vi "Support_CheckLogCallOrder.vi"(2 "log":T1[](array[typedef]) {"timestamp" format="%<%H:%M:%S%2u\n%Y/%m/%d>T"}, 3 "Wanted call order VIs":string[](array[string]), 5 "error in (no error)":errorcluster, 7 "start index":i32, 9 "length":i32=-1) -> (16 "Correct call order?":bool, 19 "error out":errorcluster)   [LabVIEW 2009]
doc: "Checks if wanted call order is same as logged call order."
uses:
  Support_LogType.ctl
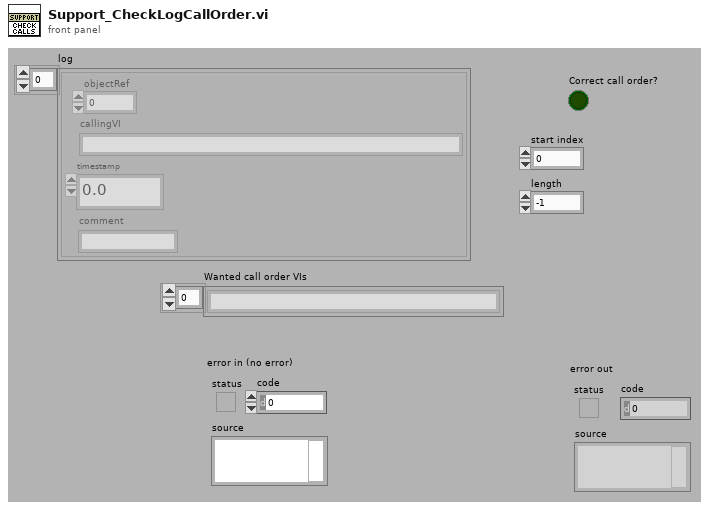
[diagram p1: front panel]
types:
  T1 = typedef "Support_LogType.ctl" = cluster{"objectRef":i32, "callingVI":string, "timestamp":dbl, "comment":string}
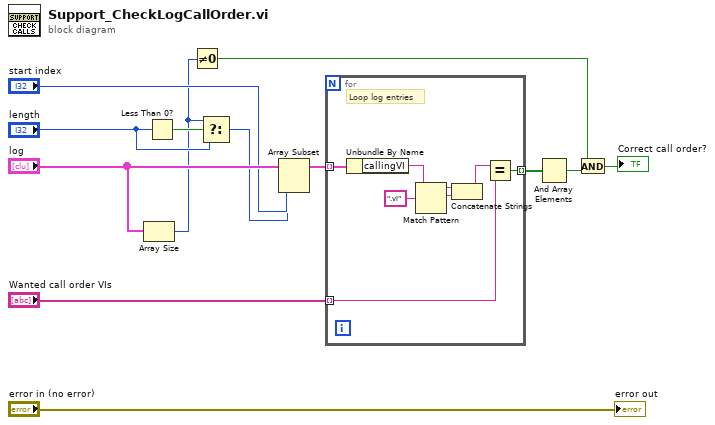
[diagram p0: block diagram]
diagram:
  n1 = Array Size(array="log") -> (size(s)=w4:i32)
  n2 = Less Than 0?(x="length") -> (x < 0?=w10:bool)
  n3 = Not Equal To 0?(x=w4) -> (x != 0?=w1:bool)
  n4 = Select(t=w4, s=w10, f="length") -> (s? t:f=w5:i32)
  n5 = Array Subset(array="log", index="start index", length=w5) -> (w8:T1[])
  n6 = for {
    tunnel: w8 -> [w21] mode=indexing
    tunnel: "Wanted call order VIs" -> [w20] mode=indexing
    tunnel: [w19] -> w11 mode=indexing
    # "Loop log entries"
    n7 = Unbundle By Name(w21) -> ("callingVI"=w18:string)
    n8 = Match Pattern(string=w18, regular expression=".vi") -> (before substring=w16:string, match substring=w15:string)  [unwired: 1 in, 2 out]
    n9 = Concatenate Strings(w16, w15) -> (w14:string)
    n10 = Equal?(x=w14, y=w20) -> (x = y?=w19:bool)
  }
  n11 = And Array Elements(Boolean array=w11) -> (logical AND=w3:bool)
  n12 = And(x=w1, y=w3) -> (x .and. y?=→"Correct call order?":bool)
  "error out" <- "error in (no error)"
